vi "Bug2 Initialize.vi"(8 "error in (no error)":errorcluster, 9 "goal reference":refnum<data-value>, 10 "start reference":refnum<data-value>, 11 "map reference out":refnum<data-value>) -> (0 "error out":errorcluster, 3 "RVCLibrary_Bug2 out":refnum<class "RVCLibrary_Bug2.lvclass">)   [LabVIEW 2013, in "RVCLibrary_Bug2.lvclass"]
uses:
  RVCLibrary_Bug2.lvclass
  <vilib>/robotics/Navigation/shared/MapNode/AbstractDstarNode/NI_Robotics_AbstractDstarNode.lvclass
  <vilib>/robotics/Navigation/shared/WorldMap/OccupancyGridWorldMap/NI_Robotics_OccupancyGridWorldMap.lvclass
  RVCLibrary_Bug2.lvclass/RVCLibrary_Bug2.ctl
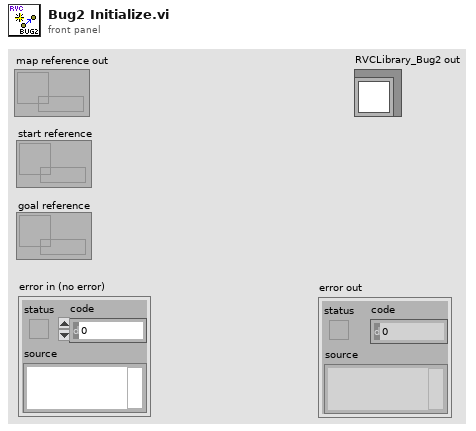
[diagram p1: front panel]
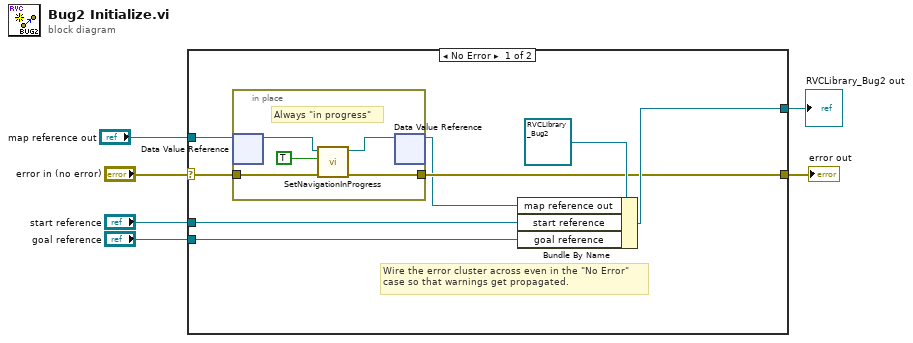
[diagram p0: block diagram]
diagram:
  n1 = case shown="No Error" "error in (no error)" {
    selector: "error in (no error)" -> [w14 w20]
    tunnel: [w9 w20] -> w5
    tunnel: "map reference out" -> [w8 _]
    tunnel: "start reference" -> [w12 _]
    tunnel: "goal reference" -> [w11 _]
    tunnel: [w10 _] -> w2
    frame No Error {
      # "Wire the error cluster across even in the \"No Error\"\ncase so that warnings get propagated."
      n2 = in-place {
        in-place-border: [w16] -> w9
        in-place-border: w14 -> [w15]
        # "Always \"in progress\""
        n3 = in-place-dvr #1(w8) -> (w19:refnum<class "NI_Robotics_OccupancyGridWorldMap.lvclass">)  [unwired: 1 out]
        n4 = call-dynamic "SetNavigationInProgress.vi"("error in (no error)"=w15, "navigation in progress"=TRUE ("Navigation in Progress"), "AbstractWorldMap in"=w19) -> ("error out"=w16:errorcluster, "AbstractWorldMap out"=w17:refnum<class "NI_Robotics_OccupancyGridWorldMap.lvclass">)  [unwired: 7 in]
        n5 = in-place-dvr #1(w17) -> (w7:refnum<data-value>)  [unwired: 1 out]
      }
      n6 = Bundle By Name(cluster=refnum<class "RVCLibrary_Bug2.lvclass"> refnum ("RVCLibrary_Bug2.lvclass"), "map reference out"=w7, "start reference"=w12, "goal reference"=w11) -> (w10:refnum<class "RVCLibrary_Bug2.lvclass">)
    }
    frame Error {
    }
  }
  "error out" <- w5
  "RVCLibrary_Bug2 out" <- w2
